vi "Interface.vi"() -> ()   [LabVIEW 2011]
doc: "This example shows how to capture and display an image from a grab acquisition\n\nSteps to run:\n\n1. Ensure interface name is correct for your camera and system setup\n2. Run the VI\n3. When you want to capture an image click the Get Image control."
uses:
  <vilib>/userdefined/High Color/IMAQdx.ctl
  <vilib>/vision/driver/NI_Vision_Acquisition_Software.lvlib
panel:
  in  "Camera":T1
  in  "stop":bool
  in  "Get Image":bool
  out "Snap Image":T2(plugin-control)
  out "Grab Image":T2(plugin-control)
  # "Note: You must have IMAQdx installed\nto run this example."
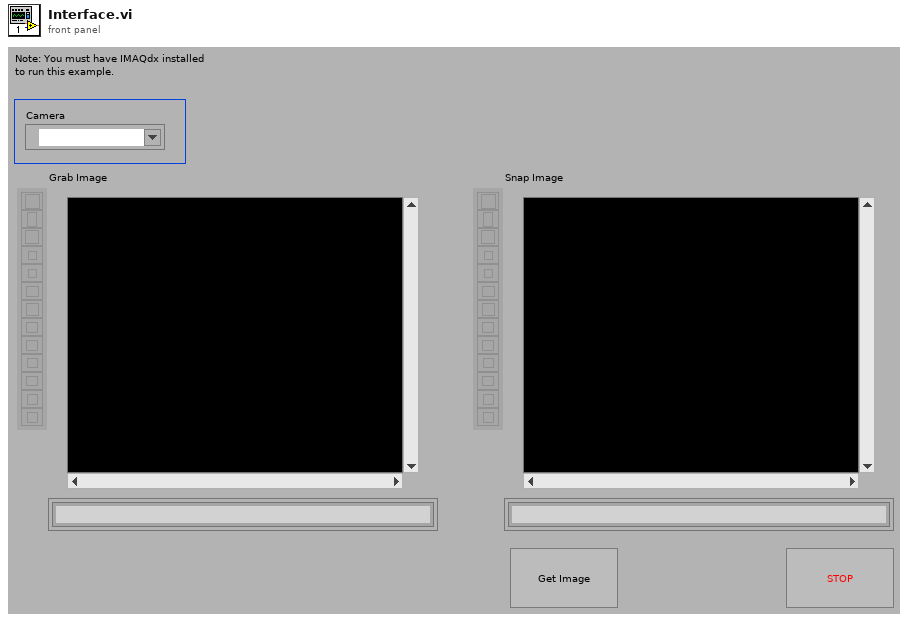
[diagram p1: front panel]
types:
  T1 = typedef "IMAQdx.ctl" = refnum<k21>
  T2 = typedef "IMAQ Image.ctl" = refnum<image>
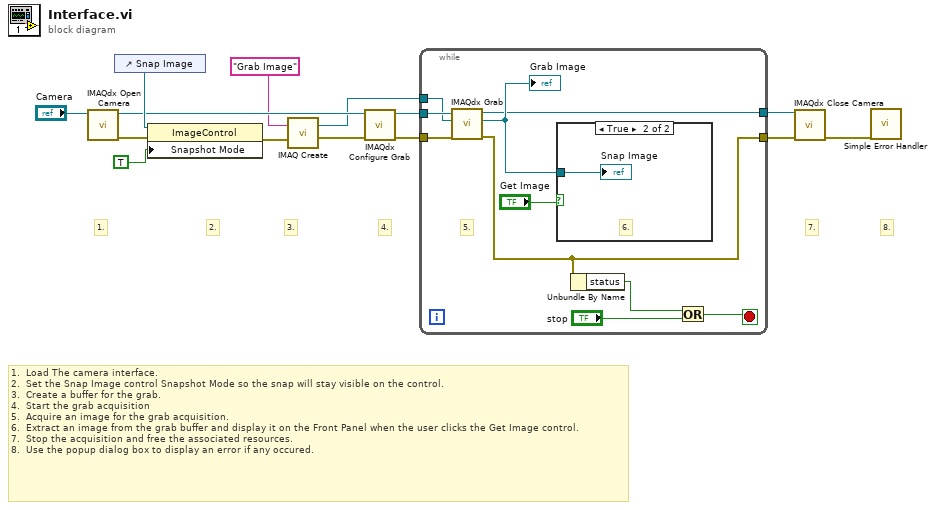
[diagram p0: block diagram]
diagram:
  # "8."
  # "7."
  # "4."
  # "3."
  # "2."
  # "1."
  # "1.  Load The camera interface.\n2.  Set the Snap Image control Snapshot Mode so the snap will stay visible on the control.\n3.  Create a buffer for the grab.\n4.  Start the grab acquisition\n5.  Acquire an image for the grab acquisition.\n6.  Extract an image from the grab buffer and display it on the Front Panel when the user clicks the Get Image control.\n7.  Stop the acquisition and free the associated resources.\n8.  Use the popup dialog box to display an error if any occured."
  n1 = call <vilib>:"IMAQdx Open Camera.vi"("Session In"="Camera") -> ("error out"=w13:errorcluster, "Session Out"=w12:T1)  [unwired: 2 in, 7 out]
  n2 = control-ref of="Snap Image"() -> (w14:refnum<vi>)
  n3 = property class="ImageControl"(reference=w14, error in=w13, "Snapshot Mode"=TRUE) -> (error out=w9:errorcluster)  [unwired: 1 out]
  n4 = call "IMAQ Create"("Image Name"="Grab Image", "error in (no error)"=w9) -> ("New Image"=w7:T2, "error out"=w8:errorcluster)  [unwired: 2 in, 1 out]
  n5 = call <vilib>:"IMAQdx Configure Grab.vi"("error in"=w8, "Session In"=w12) -> ("error out"=w6:errorcluster, "Session Out"=w11:T1)  [unwired: 8 out]
  n6 = while {
    tunnel: w11 -> [w22]
    tunnel: [w21] -> w10
    tunnel: w7 -> [w20]
    tunnel: w6 -> [w19]
    tunnel: [w18] -> w5
    stop <- w15 stop-if-true
    # "5."
    n7 = call <vilib>:"IMAQdx Grab.vi"("error in"=w19, "Image In"=w20, "Session In"=w22) -> ("error out"=w18:errorcluster, "Image Out"=w23:T2, "Session Out"=w21:T1)  [unwired: 1 in, 5 out]
    "Grab Image" <- w23
    n8 = case shown="True" "Get Image" {
      tunnel: w23 -> [_ w25]
      frame False {
      }
      frame True {
        # "6."
        "Snap Image" <- w25
      }
    }
    n9 = Unbundle By Name(w18) -> ("status"=w17:bool)
    n10 = Or(x=w17, y="stop") -> (x .or. y?=w15:bool)
  }
  n11 = call <vilib>:"IMAQdx Close Camera.vi"("error in"=w5, "Session In"=w10) -> ("error out"=w3:errorcluster)  [unwired: 9 out]
  n12 = call <vilib>:"Simple Error Handler.vi"("error in (no error)"=w3) -> ()  [unwired: 1 in, 8 out]
